vi "Configure Serial Input Active Lane Count.vi"(0 "fpga interface in":refnum<k20>, 5 "serial input channels":string[](array[string]), 7 "serial input active lane counts":i32[](array[ring])=[4] items=["1 Lane"=1, "2 Lanes"=2, "4 Lanes"=4], 11 "error in (no error)":errorcluster) -> (4 "fpga interface out":refnum<k20>, 15 "error out":errorcluster)   [LabVIEW 2023, in "GettingStarted_Common_148X_Host.lvlib"]
uses:
  GettingStarted_Common_148X_Host.lvlib
  <instrlib>/FlexRIO/API/Host/v1/NI FlexRIO/API/Get Property Reference - Fpga Small.vi
  <resource>/objmgr/niflexrioapiChannel.rc
  <instrlib>/FlexRIO/API/Host/v1/NI FlexRIO API v1.lvlib
  <resource>/objmgr/niflexrioapi.rc
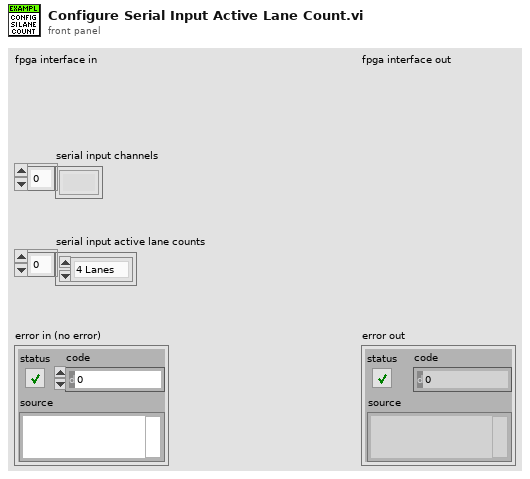
[diagram p1: front panel]
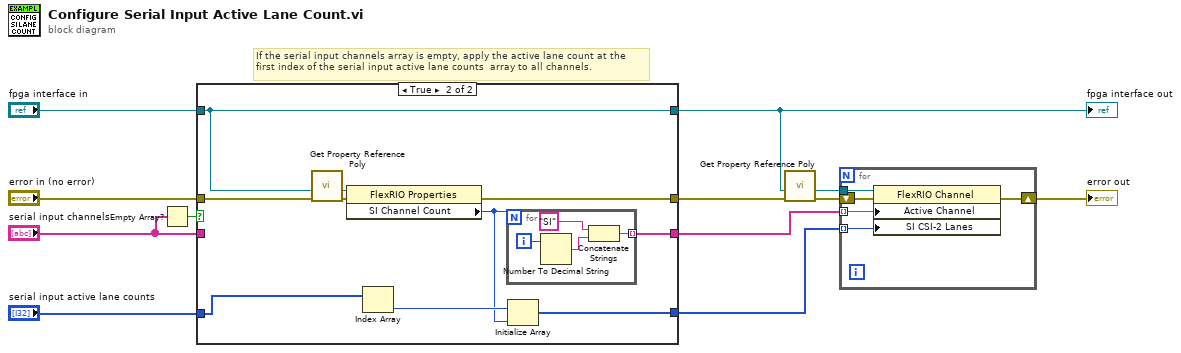
[diagram p0: block diagram]
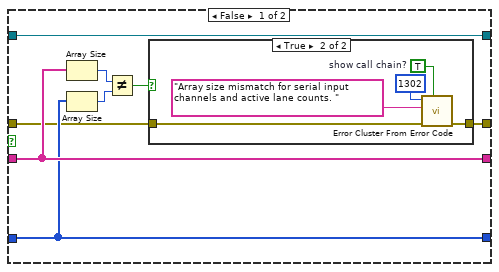
[diagram p2: hidden frame]
diagram:
  # "If the serial input channels array is empty, apply the active lane count at the first index of the serial input active lane counts  array to all channels."
  n1 = Empty Array?(array="serial input channels") -> (empty?=w4:bool)
  n2 = case shown="True" w4 {
    tunnel: "serial input channels" -> [w19 _]
    tunnel: "error in (no error)" -> [w14 w33]
    tunnel: [w19 w34] -> w6
    tunnel: "fpga interface in" -> [w20 w32]
    tunnel: [w20 w32] -> w8
    tunnel: [w13 w31] -> w7
    tunnel: [w18 w29] -> w1
    tunnel: "serial input active lane counts" -> [w18 w28]
    frame False {
      n3 = Array Size(array=w19) -> (size(s)=w16:i32)
      n4 = Array Size(array=w18) -> (size(s)=w17:i32)
      n5 = Not Equal?(x=w16, y=w17) -> (x != y?=w15:bool)
      n6 = case shown="True" w15 {
        tunnel: [w21 w22] -> w13
        tunnel: w14 -> [w21 w23]
        frame False {
        }
        frame True {
          w24 = TRUE  # show call chain?
          n7 = call <vilib>:"Error Cluster From Error Code.vi"("show call chain? (False)"=w24, "error in (no error)"=w23, "error message (\"\")"="Array size mismatch for serial input channels and active lane counts. ", "error code (0)"=1302) -> ("error out"=w22:errorcluster)  [unwired: 5 in]
        }
      }
    }
    frame True {
      n8 = call-poly <instrlib>:"Get Property Reference Poly.vi"("error in (no error)"=w33, "fpga interface in"=w32) -> ("error out"=w35:errorcluster, "property reference"=w36:refnum<k20>)  [unwired: 4 in, 1 out]
      n9 = property class="FlexRIO Properties"(reference=w36, error in=w35) -> (error out=w31:errorcluster, "SI Channel Count"=w27:i32)  [unwired: 1 out]
      n10 = Index Array(array=w28) -> (element=w30:i32)  [unwired: 1 in]
      n11 = for {
        N: w27 -> [_]
        tunnel: [w37] -> w34 mode=indexing
        i -> [w40]
        n12 = Number To Decimal String(number=w40) -> (decimal integer string=w39:string)  [unwired: 1 in]
        n13 = Concatenate Strings("SI", w39) -> (w37:string)
      }
      n14 = Initialize Array(w30, w27) -> (w29:i32[])
    }
  }
  "fpga interface out" <- w8
  n15 = call-poly <instrlib>:"Get Property Reference Poly.vi"("error in (no error)"=w7, "fpga interface in"=w8) -> ("error out"=w12:errorcluster, "property reference"=w11:refnum<k20>)  [unwired: 4 in, 1 out]
  n16 = for {
    tunnel: w11 -> [w44]
    shift-right: [w43] -> w10
    shift-left: w12 -> [w45]
    tunnel: w6 -> [w42] mode=indexing
    tunnel: w1 -> [w41] mode=indexing
    n17 = property class="FlexRIO Channel"(reference=w44, error in=w45, "Active Channel"=w42, "SI CSI-2 Lanes"=w41) -> (error out=w43:errorcluster)  [unwired: 1 out]
  }
  "error out" <- w10
